vi "for_v0_v6.vi"() -> ()   [LabVIEW 2009]
uses:
  <vilib>/Platform/portaccess.llb/Out Port8.vi
panel:
  out "Numarul de iteratii":dbl=60.0
  in  "stop_while":bool
  in  "Stop_for":bool
  in  "Slide":u8(slide)=60 scale=0.0..255.0
  out "Numeric":dbl=59.0
  out "Array":bool[](array[boolean])=[FALSE, FALSE, TRUE, TRUE, TRUE, FALSE, TRUE, TRUE]
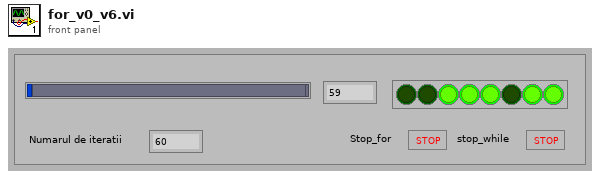
[diagram p1: front panel]
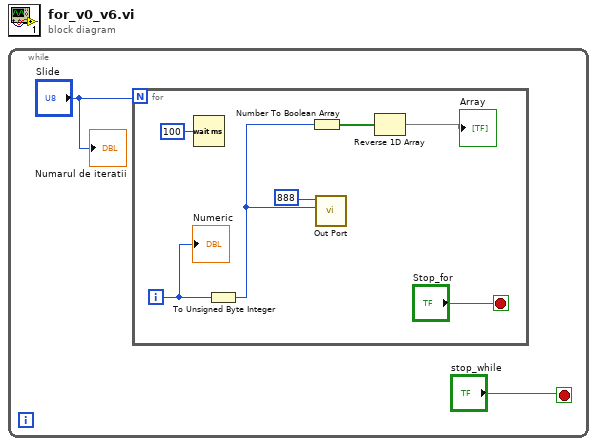
[diagram p0: block diagram]
diagram:
  n1 = while {
    stop <- "stop_while" stop-if-true
    n2 = for {
      N: "Slide" -> [_]
      i -> [w4]
      stop <- "Stop_for" stop-if-true
      n3 = Wait (ms)(milliseconds to wait=u32 100) -> ()  [unwired: 1 out]
      n4 = To Unsigned Byte Integer(number=w4) -> (unsigned 8bit integer=w5:u8)
      n5 = Number To Boolean Array(number=w5) -> (Boolean array=w9:bool[])
      n6 = call-poly <vilib>:"Out Port.vi"("write value"=w5, "address"=888) -> ()  [unwired: 7 in, 1 out]
      n7 = Reverse 1D Array(array=w9) -> (reversed array=→"Array":bool[])
      "Numeric" <- w4
    }
    "Numarul de iteratii" <- "Slide"
  }
